vi "Stop Log.vi"(8 "error in (no error)":errorcluster, 11 "DataLogger in":refnum<class "DataLogger.lvclass">) -> (0 "error out":errorcluster, 3 "DataLogger out":refnum<class "DataLogger.lvclass">)   [LabVIEW 2020, in "VolatusData.lvlib" / "DataLogger.lvclass"]
uses:
  DataLogger.lvclass
  DataLogger.lvclass/DataLogger.ctl
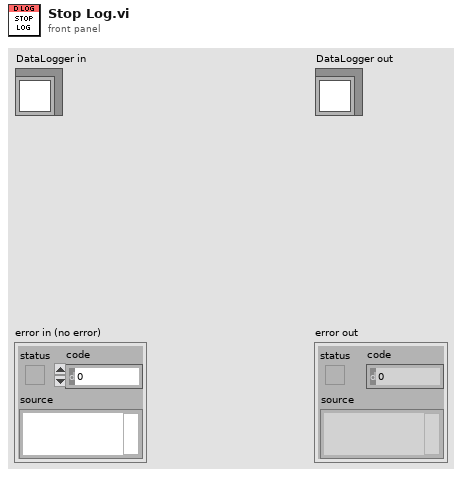
[diagram p1: front panel]
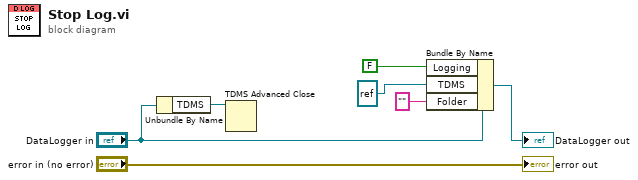
[diagram p0: block diagram]
diagram:
  n1 = Unbundle By Name("DataLogger in") -> ("TDMS"=w1:refnum<k34>)
  n2 = TDMS Advanced Close(11:w1) -> ()  [unwired: 3 in, 2 out]
  n3 = Bundle By Name(cluster="DataLogger in", "Logging"=FALSE, "TDMS"=refnum<k34> refnum, "Folder"="") -> (→"DataLogger out":refnum<class "DataLogger.lvclass">)
  "error out" <- "error in (no error)"
